vi "VISA Interface Type.vi"(8 "error in (no error)":errorcluster, 11 "VISA in":refnum<visa-resource-name>) -> (0 "error out":errorcluster, 2 "Interface Type":T1(ring), 3 "VISA out":refnum<visa-resource-name>)   [LabVIEW 2018]
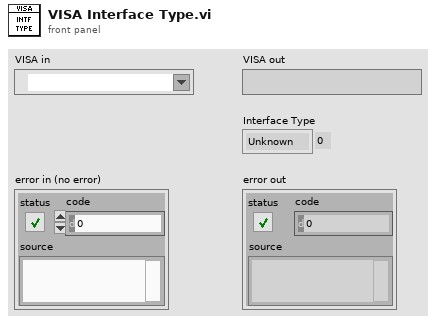
[diagram p1: front panel]
types:
  T1 = enum16{"Unknown", "GPIB", "VXI", "GPIB-VXI", "Serial", "PXI", "TCPIP", "USB", "FireWire"}
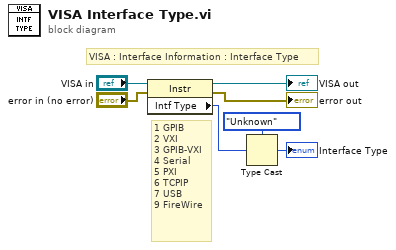
[diagram p0: block diagram]
diagram:
  # "VISA : Interface Information : Interface Type"
  # "1\tGPIB\n2\tVXI\n3\tGPIB-VXI\n4\tSerial\n5\tPXI\n6\tTCPIP\n7\tUSB\n9\tFireWire"
  n1 = property class="Instr"(reference="VISA in", error in="error in (no error)") -> (reference out=→"VISA out":refnum<visa-resource-name>, error out=→"error out":errorcluster, "Intf Type"=w5:u16)
  n2 = Type Cast(type=T1."Unknown" ("Interface Type"), x=w5) -> (*(type *) &x=→"Interface Type":T1)
